vi "degauss state queue.vi"(10 "daguas max current":dbl, 11 "Channel Index":i16) -> (3 "concatenated string":string)   [LabVIEW 2020, in "TDK-Lambda Z Bipolar.lvclass"]
uses:
  TDK-Lambda Z Bipolar.lvclass
panel:
  out "decimal integer string":string
  out "Setcurrent":dbl
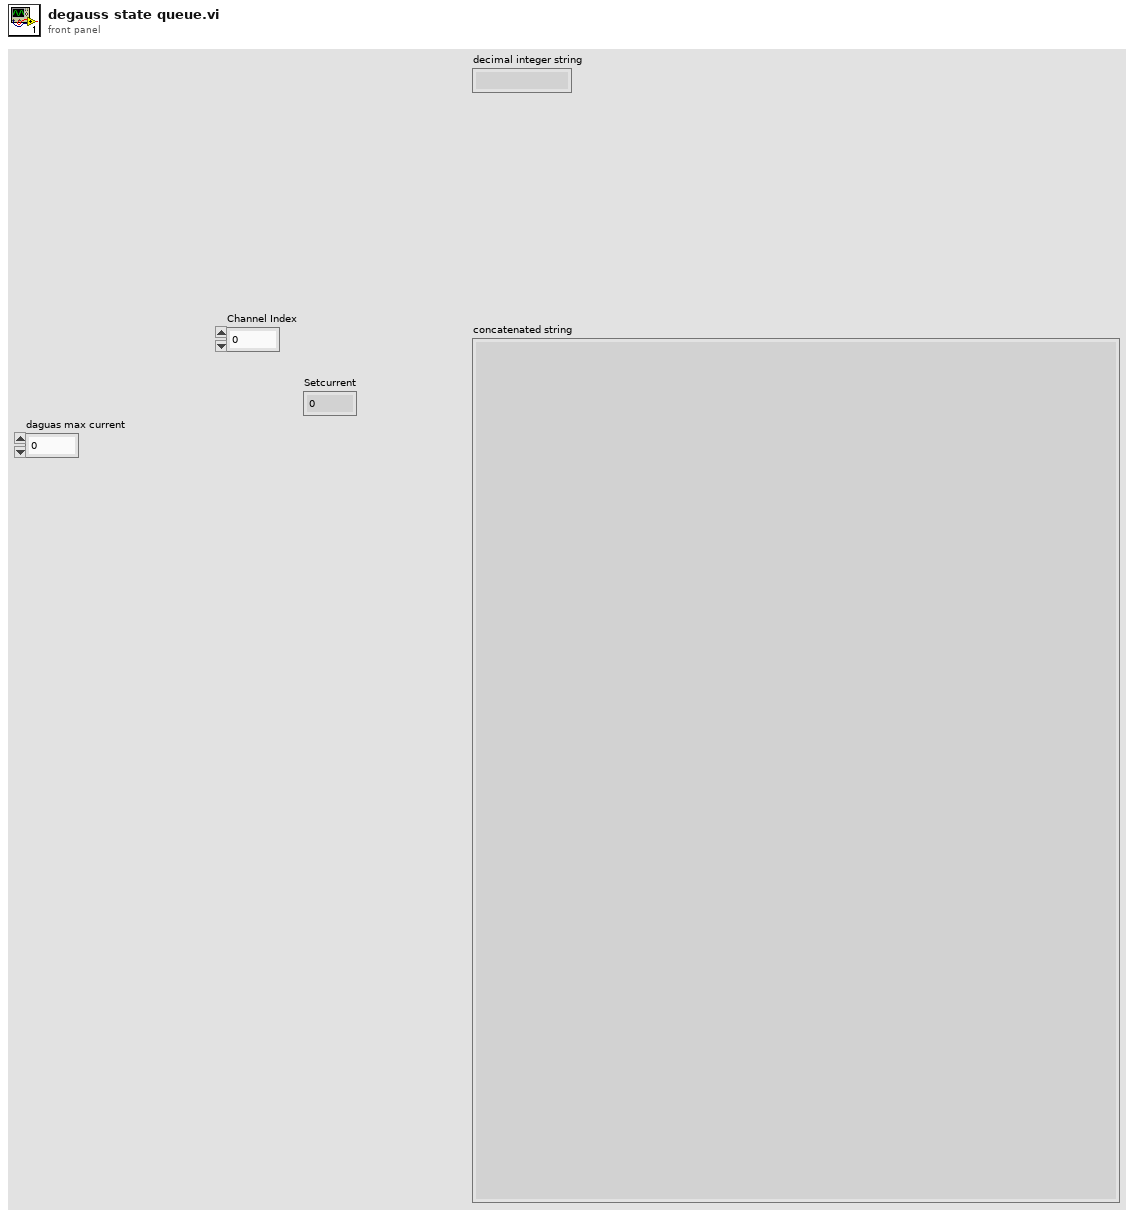
[diagram p1: front panel]
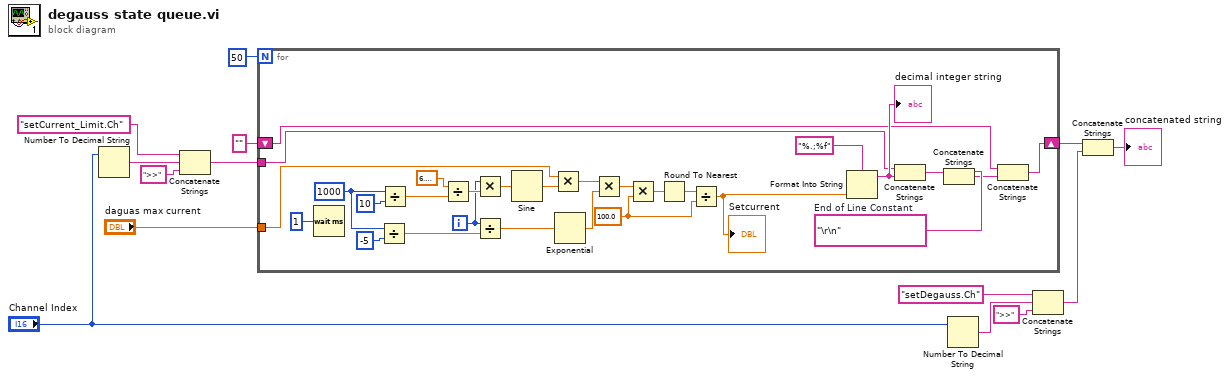
[diagram p0: block diagram]
diagram:
  n1 = Number To Decimal String(number="Channel Index") -> (decimal integer string=w9:string)  [unwired: 1 in]
  n2 = Concatenate Strings("setCurrent_Limit.Ch" ("string"), w9, ">>" ("string")) -> (w8:string)
  n3 = for {
    N: 50 -> [_]
    tunnel: "daguas max current" -> [w29]
    shift-right: [w20] -> w3
    shift-left: "" -> [w19]
    tunnel: w8 -> [w15]
    i -> [w30]
    w17 = "\r\n"  # End of Line Constant
    w22 = 100.0 ("y")
    w33 = 1000
    n4 = Wait (ms)(milliseconds to wait=u32 1) -> ()  [unwired: 1 out]
    n5 = Divide(x=w33, y=-5) -> (x/y=w39:dbl)
    n6 = Divide(x=w33, y=10) -> (x/y=w40:dbl)
    n7 = Divide(x=6.283185307179586, y=w40) -> (x/y=w35:dbl)
    n8 = Multiply(x=w30, y=w35) -> (x*y=w36:dbl)
    n9 = Divide(x=w30, y=w39) -> (x/y=w37:dbl)
    n10 = Sine(x=w36) -> (sin(x)=w41:dbl)
    n11 = Multiply(x=w29, y=w41) -> (x*y=w42:dbl)
    n12 = Exponential(1:w37) -> (0:w38:dbl)
    n13 = Multiply(x=w42, y=w38) -> (x*y=w25:dbl)
    n14 = Multiply(x=w25, y=w22) -> (x*y=w24:dbl)
    n15 = Round To Nearest(number=w24) -> (nearest integer value=w23:dbl)
    n16 = Divide(x=w23, y=w22) -> (x/y=w21:dbl)
    "Setcurrent" <- w21
    n17 = Format Into String(format string="%.;%f", w21) -> (resulting string=w26:string)  [unwired: 2 in, 1 out]
    "decimal integer string" <- w26
    n18 = Concatenate Strings(w15, w26) -> (w18:string)
    n19 = Concatenate Strings(w18, w17) -> (w16:string)
    n20 = Concatenate Strings(w19, w16) -> (w20:string)
  }
  n21 = Number To Decimal String(number="Channel Index") -> (decimal integer string=w4:string)  [unwired: 1 in]
  n22 = Concatenate Strings("setDegauss.Ch" ("string"), w4, ">>" ("string")) -> (w2:string)
  n23 = Concatenate Strings(w3, w2) -> (→"concatenated string":string)
